vi "Set.vi"(10 "Value":string, 11 "Text in":refnum<class "Text.lvclass">) -> (3 "Text out":refnum<class "Text.lvclass">)   [LabVIEW 2022 SP3, in "Conditum.lvlib" / "Columns.lvlib" / "Text.lvclass"]
uses:
  Text.lvclass
  C:/dev/lv/illuminated-g/lv-conditum/Conditum/Columns/Type/Type.lvclass
  Type/Type.lvclass/Type.ctl
  Text.lvclass/Text.ctl
  Type/Type.lvclass
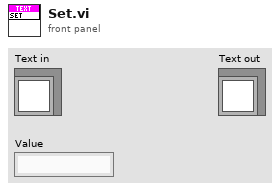
[diagram p1: front panel]
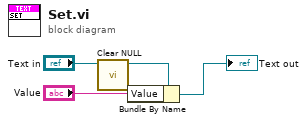
[diagram p0: block diagram]
diagram:
  n1 = call "Clear NULL.vi"("Type in"="Text in") -> ("Type out"=w1:refnum<class "Text.lvclass">)  [unwired: 10 in]
  n2 = Bundle By Name(cluster=w1, "Value"="Value") -> (→"Text out":refnum<class "Text.lvclass">)
